vi "Gain Estimator.vi"() -> ()   [LabVIEW 2015, in "SubVIs.lvlib"]
uses:
  SubVIs.lvlib
  <vilib>/Analysis/baseanly.llb/Mean (DBL).vi
  <vilib>/Analysis/NI_AALBase.lvlib
panel:
  out "Mean SPL":dbl
  out "SPL":dbl
  in  "Gain":dbl min=-50.0 max=50.0 step=1.0
  in  "Microphone Sensitvity (dBV/Pa)":dbl format="%#_13g"
  in  "stop (F)":bool
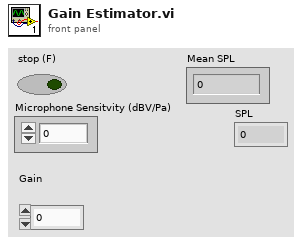
[diagram p1: front panel]
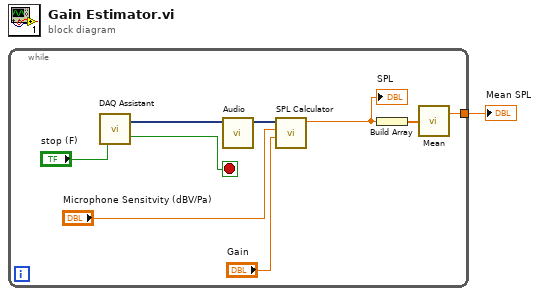
[diagram p0: block diagram]
diagram:
  n1 = while {
    tunnel: [w2] -> w1
    stop <- w9 stop-if-true
    n2 = call "DAQ Assistant"("stop (F)"="stop (F)") -> ("data"=w8:dynamicdata, "stopped"=w9:bool)  [unwired: 15 in, 2 out]
    n3 = call "Audio"("Signal"=w8) -> ("Filtered Signal"=w7:dynamicdata)  [unwired: 9 in, 1 out]
    n4 = call "SPL Calculator.vi"("Gain"="Gain", "Microphone Sensitvity (dBV/Pa)"="Microphone Sensitvity (dBV/Pa)", "Filtered Signal"=w7) -> ("SPL"=w4:dbl)  [unwired: 7 in, 1 out]
    "SPL" <- w4
    n5 = Build Array(w4) -> (w3:dbl[])
    n6 = call-poly <vilib>:"Mean.vi"("X"=w3) -> ("mean"=w2:dbl)  [unwired: 1 out]
  }
  "Mean SPL" <- w1
